vi "Get Status.vi"(0 "disk streaming in":refnum<class "Disk Streaming.lvclass">, 5 "error in (no error)":errorcluster) -> (11 "Host DMA buffer size (bytes)":u64, 13 "Disk maximum async operations":u32, 14 "disk streaming out":refnum<class "Disk Streaming.lvclass">, 15 "finished":bool, 16 "Disk pending async operations":u32, 17 "Host DMA buffer utilization (bytes)":u64, 18 "preview data":i16[](array[numeric]), 19 "error out":errorcluster)   [LabVIEW 2021, in "Disk Streaming.lvclass"]
doc: "Returns the status of a streaming process controlled by a disk streaming instance. For more information about the disk streaming instance refer to the <B>Open.vi</B> context help.\n\nInputs:\n\n<B>disk streaming in</B>: Disk streaming instance input.\n\nOutputs:\n\n<B>disk streaming out</B>: Disk streaming instance output. Pass this output to the other Disk Streaming VIs to perform the streaming.\n\n<B>finished</B>: Indicates whether the streaming is finished.\n\n<B>Disk pending async operations</B>: The number of asynchronous reads or writes that are currently running in the background.\n\n<B>Disk maximum async operations</B>: The maximum number of asynchronous reads or writes that can run simultaneously in the background.\n\n<B>Host DMA buffer utilization (bytes)</B>: The used space, in bytes, in the host DMA buffer.\n\n<B>Host DMA buffer size (bytes)</B>: The size, in bytes, of the host DMA buffer.\n\n<B>preview data</B>: Array of I16s containing the preview samples. The preview is a snapshot of the recently streamed samples, a small part of the sample sequence transferred between the disk and the FPGA Target. The preview is updated only on <B>Read</B> and <B>Write</B> VI calls, and the size of the array can be configured using the <B>Configure Status.vi</B>."
uses:
  Disk Streaming.lvclass
  Disk Streaming.lvclass/Disk Streaming.ctl
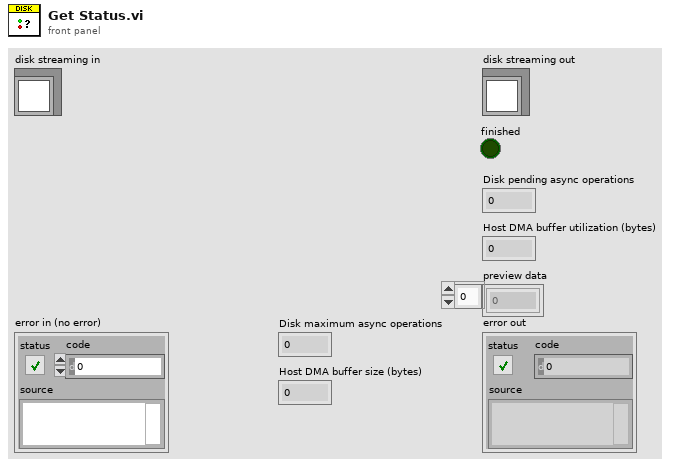
[diagram p1: front panel]
types:
  T1 = typedef "Disk Streaming.lvclass/Status.ctl" = cluster{"finished":bool, "Host DMA buffer size (bytes)":u64, "Host DMA buffer utilization (bytes)":u64, "Disk maximum async operations":u32, "Disk pending async operations":u32, "preview data":i16[]}
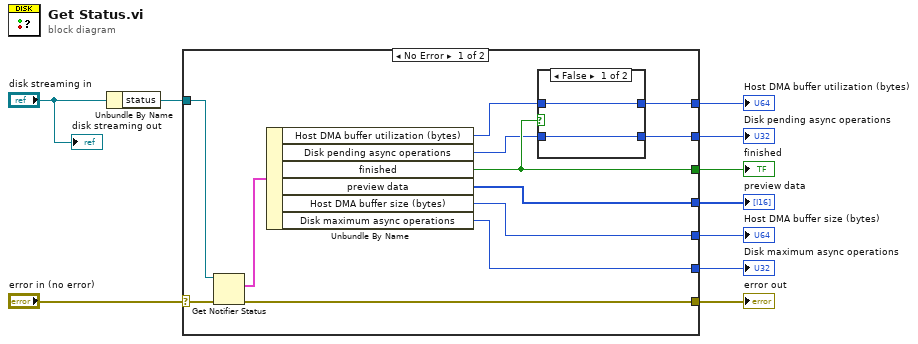
[diagram p0: block diagram]
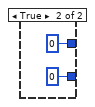
[diagram p2: hidden frame]
diagram:
  n1 = Unbundle By Name("disk streaming in") -> ("status"=w7:refnum<notifier>)
  n2 = case shown="No Error" "error in (no error)" {
    selector: "error in (no error)" -> [w22 w27]
    tunnel: [w14 w27] -> w9
    tunnel: w7 -> [w21 _]
    tunnel: [w19 _] -> w6
    tunnel: [w12 _] -> w5
    tunnel: [w17 _] -> w4
    tunnel: [w11 _] -> w3
    tunnel: [w15 _] -> w2
    tunnel: [w13 _] -> w1
    frame No Error {
      n3 = Get Notifier Status(notifier=w21, error in (no error)=w22) -> (current notification=w20:T1, error out=w14:errorcluster)  [unwired: 3 out]
      n4 = Unbundle By Name(w20) -> ("Host DMA buffer utilization (bytes)"=w18:u64, "Disk pending async operations"=w16:u32, "finished"=w19:bool, "preview data"=w13:i16[], "Host DMA buffer size (bytes)"=w12:u64, "Disk maximum async operations"=w11:u32)
      n5 = case shown="False" w19 {
        tunnel: w18 -> [w24 _]
        tunnel: [w24 u64 0 ("Host DMA buffer utilization (bytes)")] -> w17
        tunnel: w16 -> [w23 _]
        tunnel: [w23 u32 0 ("Disk pending async operations")] -> w15
        frame False {
        }
        frame True {
        }
      }
    }
    frame Error {
    }
  }
  "error out" <- w9
  "preview data" <- w1
  "finished" <- w6
  "Host DMA buffer size (bytes)" <- w5
  "Host DMA buffer utilization (bytes)" <- w4
  "Disk maximum async operations" <- w3
  "Disk pending async operations" <- w2
  "disk streaming out" <- "disk streaming in"
